vi "Set_WavelengthPower.vi"(6 "Index":u8, 8 "error in (no error)":errorcluster, 9 "Power":dbl, 10 "Wavelength":dbl[unit], 11 "NKT in":refnum<class "NKT_Extreme.lvclass">) -> (0 "error out":errorcluster, 3 "NKT out":refnum<class "NKT_Extreme.lvclass">)   [LabVIEW 2020, in "NKT_Extreme.lvclass"]
uses:
  <instrlib>/Classes/Laser/NKT/NKT_Extreme.lvclass
  <instrlib>/NKTP_API/NKTP_API.lvlib
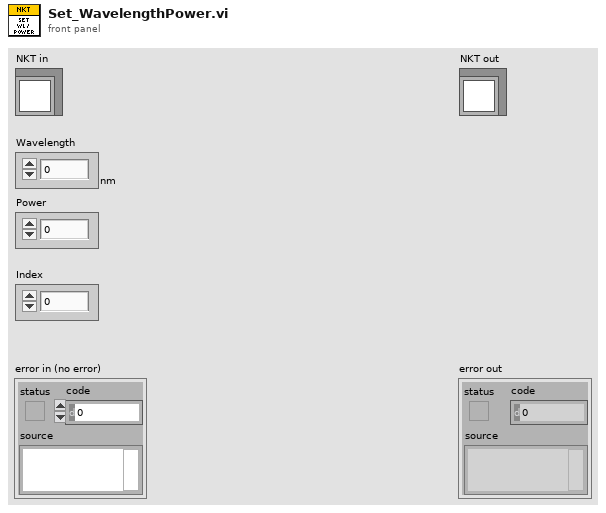
[diagram p1: front panel]
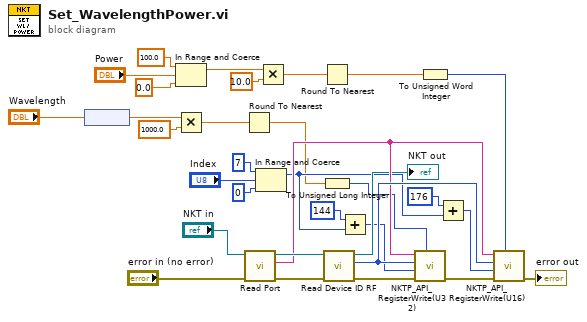
[diagram p0: block diagram]
diagram:
  n1 = node("Wavelength") -> (w5:dbl)
  n2 = In Range and Coerce(upper limit=100.0, x="Power", lower limit=0.0) -> (coerced(x)=w30:dbl)  [unwired: 1 out]
  n3 = Multiply(x=w5, y=1000.0) -> (x*y=w3:dbl)
  n4 = Round To Nearest(number=w3) -> (nearest integer value=w2:dbl)
  n5 = call-dynamic "Read Port.vi"("error in (no error)"="error in (no error)", "NKT in"="NKT in") -> ("error out"=w17:errorcluster, "Port"=w14:string, "NKT out"=w18:refnum<class "NKT_Extreme.lvclass">)  [unwired: 7 in]
  n6 = In Range and Coerce(upper limit=u8 7, x="Index", lower limit=u8 0) -> (coerced(x)=w8:u8)  [unwired: 1 out]
  n7 = Multiply(x=w30, y=10.0) -> (x*y=w28:dbl)
  n8 = Round To Nearest(number=w28) -> (nearest integer value=w27:dbl)
  n9 = To Unsigned Long Integer(number=w2) -> (unsigned 32bit integer=w1:u32)
  n10 = call-dynamic "Read Device ID RF.vi"("error in (no error)"=w17, "NKT in"=w18) -> ("error out"=w13:errorcluster, "Device ID RF"=w15:u8, "NKT out"=→"NKT out":refnum<class "NKT_Extreme.lvclass">)  [unwired: 7 in]
  n11 = Add(x=u8 144 ("regId"), y=w8) -> (x+y=w7:u8)
  n12 = call <instrlib>:"NKTP_API_RegisterWrite(U32).vi"("value"=w1, "error in"=w13, "regId"=w7, "devId"=w15, "portname"=w14) -> ("error out"=w12:errorcluster)  [unwired: 5 in, 1 out]
  n13 = To Unsigned Word Integer(number=w27) -> (unsigned 16bit integer=w25:u16)
  n14 = Add(x=u8 176 ("regId"), y=w8) -> (x+y=w20:u8)
  n15 = call <instrlib>:"NKTP_API_RegisterWrite(U16).vi"("value"=w25, "error in"=w12, "regId"=w20, "devId"=w15, "portname"=w14) -> ("error out"=→"error out":errorcluster)  [unwired: 5 in, 1 out]
